vi "InitResultFile.vi"(8 "error in (no error)":errorcluster, 11 "PmuAnalysis in":refnum<class "PmuAnalysis.lvclass">) -> (0 "error out":errorcluster, 3 "PmuAnalysis out":refnum<class "PmuAnalysis.lvclass">)   [LabVIEW 2018, in "AnalysisPlugins.lvlib" / "PmuAnalysis.lvclass"]
uses:
  PmuAnalysis.lvclass
  X:/Projects/PMUCal/Modules/Analysis/AnalysisPlugins/AnalysisPluginBaseClass/AnalysisPluginsBase.lvclass
  FGen/MemberClasses/PmuTestFunctions/Typedefs/PmuTestParams.ctl
  FGen/MemberClasses/PmuTestFunctions/Typedefs/eParamIdx.ctl
  AnalysisPluginBaseClass/AnalysisPluginsBase.lvclass/AnalysisPluginsBase.ctl
  AnalysisPluginBaseClass/Accessors/Read ResultPath.vi
  AnalysisPluginBaseClass/Accessors/Read FileName.vi
  <vilib>/Utility/file.llb/Write Delimited Spreadsheet (string).vi
  FGen/MemberClasses/PmuTestFunctions/PmuTestFunctions.lvclass
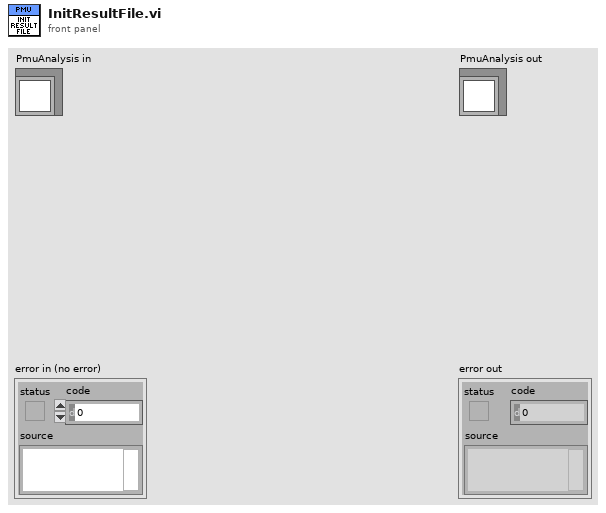
[diagram p1: front panel]
types:
  T1 = typedef "Functions.lvlib/PmuTestFunctions.lvclass/PmuTestParams.ctl" = dbl[][]
  T2 = typedef "Functions.lvlib/PmuTestFunctions.lvclass/eParamIdx.ctl" = enum16{"Xm", "Fin", "Ps", "Fh", "Ph", "Kh", "Fa", "Ka", "Fx", "Kx", "Rf", "KaS", "KxS", "KfS", "KrS"}
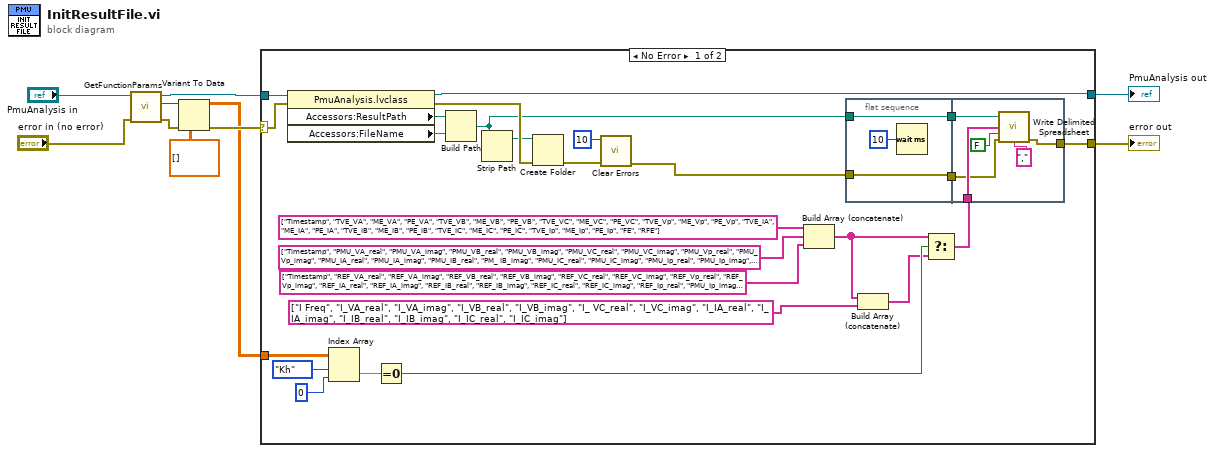
[diagram p0: block diagram]
diagram:
  n1 = call-dynamic "GetFunctionParams.vi"("error in (no error)"="error in (no error)", "PmuAnalysis in"="PmuAnalysis in") -> ("error out"=w3:errorcluster, "FunctionParams"=w5:variant, "PmuAnalysis out"=w4:refnum<class "PmuAnalysis.lvclass">)  [unwired: 7 in]
  n2 = Variant To Data(error in=w3, type=T1 [] ("Accessors:PmuTestParams"), Variant=w5) -> (data=w1:T1, error out=w2:errorcluster)
  n3 = case shown="No Error" w2 {
    selector: w2 -> [w35 w47]
    tunnel: [w22 w47] -> w10
    tunnel: w4 -> [w36 w46]
    tunnel: [w27 w46] -> w9
    tunnel: w1 -> [w19 _]
    frame No Error {
      n4 = property class="PmuAnalysis.lvclass"(reference=w36, error in=w35) -> (reference out=w27:refnum<class "PmuAnalysis.lvclass">, error out=w31:errorcluster, "Accessors:ResultPath"=w25:path, "Accessors:FileName"=w26:string)
      n5 = Index Array(array=w19, index (row)=eParamIdx."Kh" ("eParamIdx"), index (col)=0 ("disabled index (col)")) -> (element=w16:dbl)
      n6 = Equal To 0?(x=w16) -> (x = 0?=w15:bool)
      n7 = Build Path(base path=w25, name or relative path=w26) -> (appended path=w20:path)
      n8 = Strip Path(path=w20) -> (stripped path=w21:path)  [unwired: 1 out]
      n9 = Create Folder(path (use dialog)=w21, error in=w31) -> (error out=w29:errorcluster)  [unwired: 1 in, 2 out]
      n10 = call <vilib>:"Clear Errors.vi"("error in (no error)"=w29, "specific error code to clear (0: all)"=10) -> ("error out"=w28:errorcluster)  [unwired: 4 in, 1 out]
      n11 = Build Array (concatenate)(string[] ["Timestamp", "TVE_VA", "ME_VA", "PE_VA", "TVE_VB", "ME_VB", "PE_VB", "TVE_VC", "ME_VC", "PE_VC", "TVE_Vp", "ME_Vp", "PE_Vp", "TVE_IA", "ME_IA", "PE_IA", "TVE_IB", "ME_IB", "PE_IB", "TVE_IC", "ME_IC", "PE_IC", "TVE_Ip", "ME_Ip", "PE_Ip", "FE", "RFE"], string[] ["Timestamp", "PMU_VA_real", "PMU_VA_imag", "PMU_VB_real", "PMU_VB_imag", "PMU_VC_real", "PMU_VC_imag", "PMU_Vp_real", "PMU_Vp_imag", "PMU_IA_real", "PMU_IA_imag", "PMU_IB_real", "PM_ IB_imag", "PMU_IC_real", "PMU_IC_imag", "PMU_Ip_real", "PMU_Ip_imag", "PMU_FREQ", "PMU_ROCOF"], string[] ["Timestamp", "REF_VA_real", "REF_VA_imag", "REF_VB_real", "REF_VB_imag", "REF_VC_real", "REF_VC_imag", "REF_Vp_real", "REF_Vp_imag", "REF_IA_real", "REF_IA_imag", "REF_IB_real", "REF_IB_imag", "REF_IC_real", "REF_IC_imag", "REF_Ip_real", "PMU_Ip_imag", "REF_FREQ", "REF_ROCOF"]) -> (w14:string[])
      n12 = flat-sequence {
        tunnel: w28 -> [w39]
        tunnel: w20 -> [w37]
        tunnel: [w39] -> w24
        tunnel: [w37] -> w23
        tunnel: w24 -> [w41]
        tunnel: w23 -> [w43]
        tunnel: w11 -> [w42]
        tunnel: [w40] -> w22
        frame #0 {
          n13 = Wait (ms)(milliseconds to wait=u32 10) -> ()  [unwired: 1 out]
        }
        frame #1 {
          n14 = call-poly <vilib>:"Write Delimited Spreadsheet.vi"("file path (dialog if empty)"=w43, "1D data"=w42, "append to file? (new file:F)"=FALSE, "error in (no error)"=w41, "delimiter (\\t)"="," ("delimiter (\\t)")) -> ("error out"=w40:errorcluster)  [unwired: 9 in, 1 out]
        }
      }
      n15 = Build Array (concatenate)(w14, string[] ["I Freq", "I_VA_real", "I_VA_imag", "I_VB_real", "I_VB_imag", "I_ VC_real", "I_VC_imag", "I_IA_real", "I_IA_imag", "I_IB_real", "I_IB_imag", "I_IC_real", "I_IC_imag"]) -> (w12:string[])
      n16 = Select(t=w14, s=w15, f=w12) -> (s? t:f=w11:string[])
    }
    frame Error {
    }
  }
  "error out" <- w10
  "PmuAnalysis out" <- w9
